vi "GetCalChannels.vi"(11 "Sensor Info":string[][](array[string])) -> (1 "Offsets":dbl[](array[numeric]), 2 "Slopes":dbl[](array[numeric]), 3 "CalChannels":string[](array[string]))   [LabVIEW 2018, in "Controller (Host).lvlib"]
uses:
  Controller (Host).lvlib
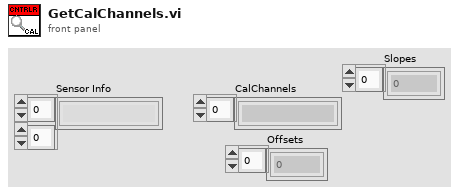
[diagram p1: front panel]
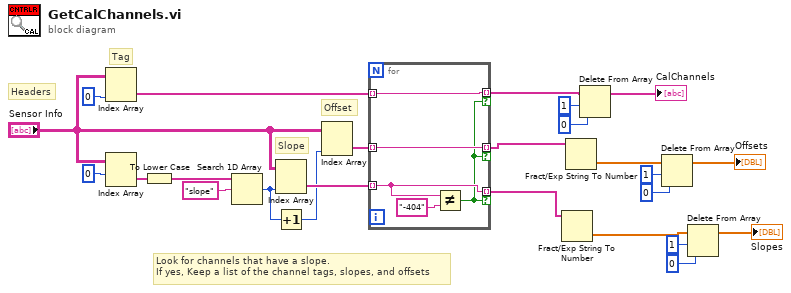
[diagram p0: block diagram]
diagram:
  # "Look for channels that have a slope. \nIf yes, Keep a list of the channel tags, slopes, and offsets"
  # "Tag"
  # "Offset"
  # "Slope"
  # "Headers"
  n1 = Index Array(array="Sensor Info", index (col)=0 ("disabled index (col)")) -> (element=w24:string[])  [unwired: 1 in]
  n2 = Index Array(array="Sensor Info", index (row)=0) -> (element=w15:string[])  [unwired: 1 in]
  n3 = To Lower Case(string=w15) -> (all lower case string=w17:string[])
  n4 = Search 1D Array(1D array=w17, element="slope") -> (index of element=w18:i32)  [unwired: 1 in]
  n5 = Index Array(array="Sensor Info", index (col)=w18) -> (element=w22:string[])  [unwired: 1 in]
  n6 = Increment(x=w18) -> (x+1=w19:i32)
  n7 = Index Array(array="Sensor Info", index (col)=w19) -> (element=w23:string[])  [unwired: 1 in]
  n8 = for {
    tunnel: w22 -> [w28] mode=indexing
    tunnel: w23 -> [w27] mode=indexing
    tunnel: w24 -> [w29] mode=indexing
    tunnel: [w29] -> w25 mode=indexing if=w26
    tunnel: [w28] -> w11 mode=indexing if=w26
    tunnel: [w27] -> w13 mode=indexing if=w26
    n9 = Not Equal?(x=w28, y="-404" ("t")) -> (x != y?=w26:bool)
  }
  n10 = Fract/Exp String To Number(string=w11) -> (number=w10:dbl[])  [unwired: 3 in, 1 out]
  n11 = Fract/Exp String To Number(string=w13) -> (number=w12:dbl[])  [unwired: 3 in, 1 out]
  n12 = Delete From Array(array=w25, length=1, index=0) -> (array with subset deleted=→"CalChannels":string[])  [unwired: 1 out]
  n13 = Delete From Array(array=w12, length=1, index=0) -> (array with subset deleted=→"Offsets":dbl[])  [unwired: 1 out]
  n14 = Delete From Array(array=w10, length=1, index=0) -> (array with subset deleted=→"Slopes":dbl[])  [unwired: 1 out]
